vi "94 BUS.vi"() -> ()   [LabVIEW 2019]
uses:
  <vilib>/httpClient/LabVIEWHTTPClient.lvlib
panel:
  out "Time Until  Bus Arrival":string
  out "Estimated Arrival Time":timestamp
  out "Current Time":string
  out "Departure Time of Bus":timestamp
  out "Current Stop Number":string
  in  "Stop Refreshing":bool
  # "Welcome to the 94 Bus!"
  # "Stop @ Intersection of College & Boston Ave."
  # "Our Stop"
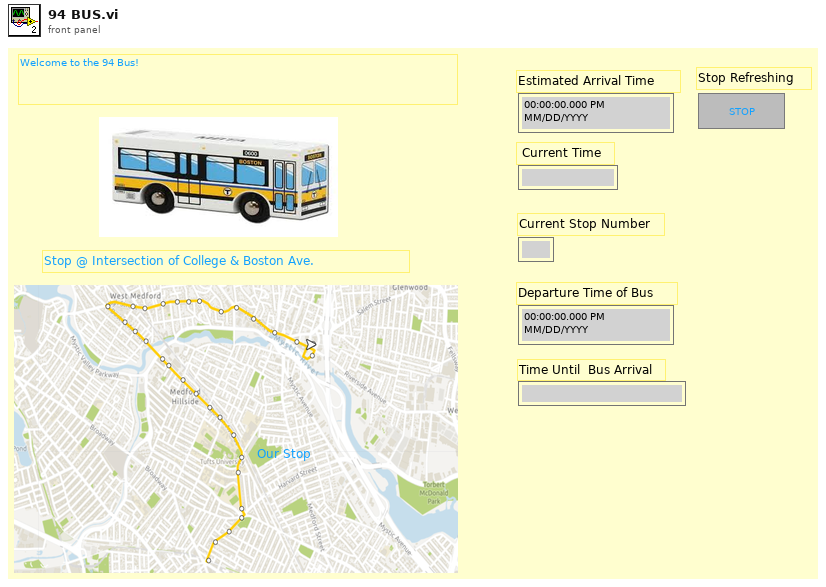
[diagram p1: front panel]
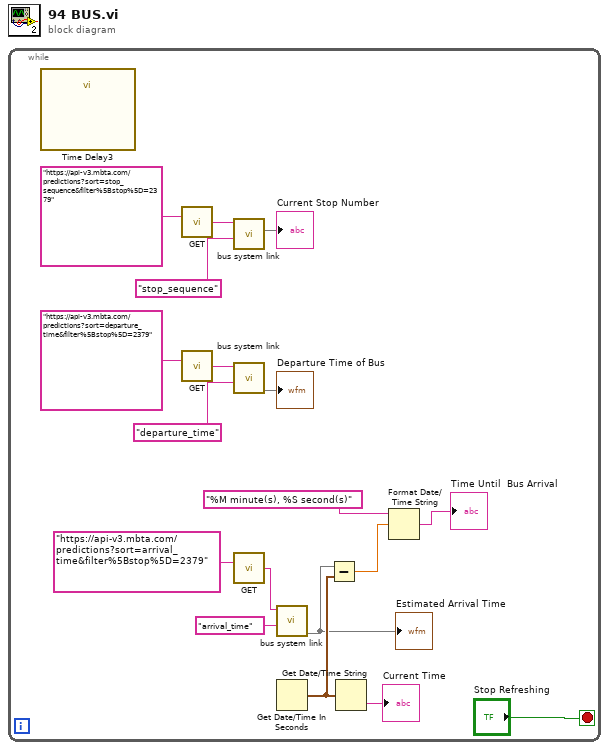
[diagram p0: block diagram]
diagram:
  n1 = while {
    stop <- "Stop Refreshing" stop-if-true
    n2 = call "Time Delay3"() -> ()  [unwired: 11 in, 1 out]
    n3 = call <vilib>:"GET.vi"("url"="https://api-v3.mbta.com/predictions?sort=stop_sequence&filter%5Bstop%5D=2379") -> ("body"=w17:string)  [unwired: 11 in, 3 out]
    n4 = call <vilib>:"GET.vi"("url"="https://api-v3.mbta.com/predictions?sort=departure_time&filter%5Bstop%5D=2379") -> ("body"=w13:string)  [unwired: 11 in, 3 out]
    n5 = call "bus system link.vi"(9:"stop_sequence" ("search name"), 11:w17) -> (2:→"Current Stop Number")  [unwired: 9 in]
    n6 = call "bus system link.vi"(9:"departure_time" ("search name"), 11:w13) -> (0:→"Departure Time of Bus")  [unwired: 9 in]
    n7 = call <vilib>:"GET.vi"("url"="https://api-v3.mbta.com/predictions?sort=arrival_time&filter%5Bstop%5D=2379") -> ("body"=w3:string)  [unwired: 11 in, 3 out]
    n8 = call "bus system link.vi"(9:"arrival_time" ("search name"), 11:w3) -> (0:w1)  [unwired: 9 in]
    "Estimated Arrival Time" <- w1
    n9 = Get Date/Time In Seconds() -> (seconds since 1Jan1904=w4:timestamp)
    n10 = Subtract(x=w1, y=w4) -> (x-y=w8:dbl)
    n11 = Get Date/Time String(seconds (now)=w4) -> (time string=→"Current Time":string)  [unwired: 2 in, 1 out]
    n12 = Format Date/Time String(time format string (%c)="%M minute(s), %S second(s)", seconds (now)=w8) -> (date/time string=→"Time Until  Bus Arrival":string)  [unwired: 1 in]
  }
